vi "MSEncoder Case-22-PhaseScan.vi"(8 "error in (no error)":errorcluster, 9 "ParamValIn":variant, 11 "MSEncoder in":refnum<class "MSEncoder.lvclass">) -> (0 "error out":errorcluster, 3 "MSEncoder out":refnum<class "MSEncoder.lvclass">)   [LabVIEW 2018, in "MSEncoder.lvclass"]
uses:
  MSEncoder.lvclass
  Ctl/MSEditorParam phaseScan.ctl
  PublicSubVI/Ctl/MathieuEqParam.ctl
  MSEncoder.lvclass/MSEncoder.ctl
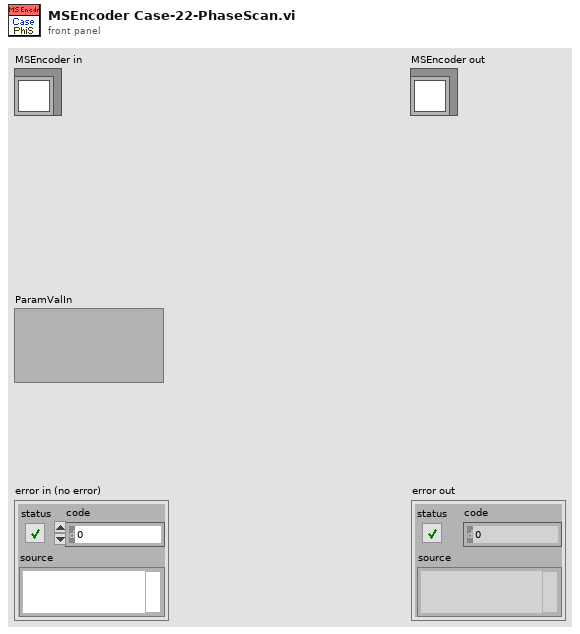
[diagram p1: front panel]
types:
  T1 = typedef "MSEditorParam phaseScan.ctl" = cluster{"auxWfmType":u32, "auxStart":u32, "iauxCyc":ext, "auxCyc":ext, "beta":ext, "betaScale":ext, "auxAmp":ext, "auxPulse1":ext[], "auxPulse2":ext[], "auxPulseAmp":ext[], "time":ext, "freq":ext[], "stepWidth":u32}
  T2 = cluster{"f1":ext, "f2":ext, "Scan Time":ext, "Stepwise":u32}
  T3 = typedef "MathieuEqParam.ctl" = cluster{"mz(Th)":ext, "Amp(V)":ext, "Freq(Hz)":ext, "Beta":ext, "r_0 (mm)":ext, "z_0 (mm)":ext}
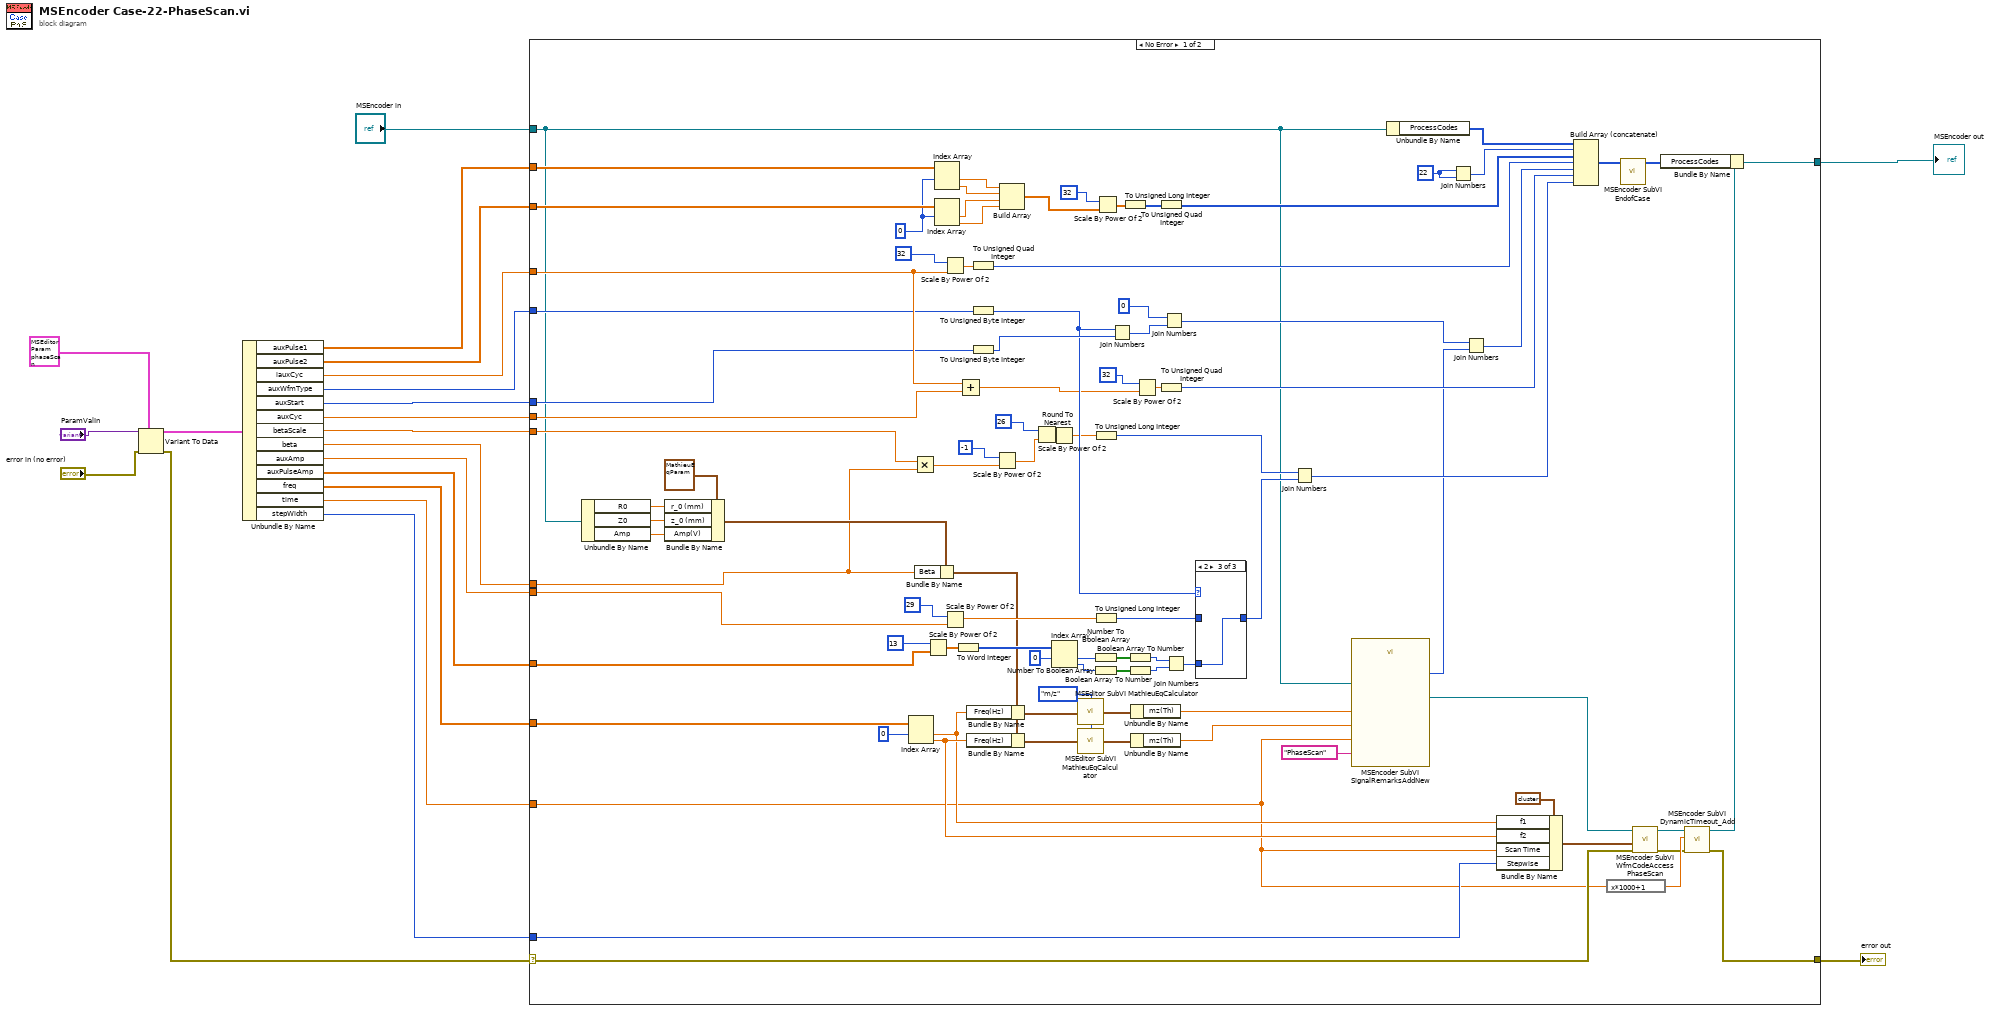
[diagram p0: block diagram]
diagram:
  n1 = Variant To Data(error in="error in (no error)", type=T1 {"auxWfmType"=0, "auxStart"=0, "iauxCyc"=0.0, "auxCyc"=0.0, "beta"=0.5, "betaScale"=1.0, "auxAmp"=1.0, "auxPulse1"=[0.0, 0.5], "auxPulse2"=[0.5, 1.0], "auxPulseAmp"=[1.0, -1.0], "time"=1.0, "freq"=[100000.0, 50000.0], "stepWidth"=1} ("ParamValueType"), Variant="ParamValIn") -> (data=w3:T1, error out=w2:errorcluster)
  n2 = Unbundle By Name(w3) -> ("auxPulse1"=w20:ext[], "auxPulse2"=w19:ext[], "iauxCyc"=w18:ext, "auxWfmType"=w17:u32, "auxStart"=w16:u32, "auxCyc"=w15:ext, "betaScale"=w14:ext, "beta"=w13:ext, "auxAmp"=w12:ext, "auxPulseAmp"=w11:ext[], "freq"=w10:ext[], "time"=w9:ext, "stepWidth"=w8:u32)
  n3 = case shown="No Error" w2 {
    selector: w2 -> [w33 w119]
    tunnel: "MSEncoder in" -> [w36 w118]
    tunnel: [w28 w119] -> w21
    tunnel: [w114 w118] -> w6
    tunnel: w20 -> [w108 _]
    tunnel: w19 -> [w107 _]
    tunnel: w18 -> [w106 _]
    tunnel: w17 -> [w105 _]
    tunnel: w16 -> [w104 _]
    tunnel: w15 -> [w103 _]
    tunnel: w14 -> [w102 _]
    tunnel: w13 -> [w101 _]
    tunnel: w12 -> [w100 _]
    tunnel: w11 -> [w99 _]
    tunnel: w10 -> [w98 _]
    tunnel: w9 -> [w27 _]
    tunnel: w8 -> [w39 _]
    frame No Error {
      w90 = u32 22
      w85 = 0 ("index")
      w93 = enum16{"m/z", "Volt", "Freq", "Beta"}."m/z" ("Target (Freq)")
      n4 = Unbundle By Name(w36) -> ("R0"=w113:ext, "Z0"=w112:ext, "Amp"=w111:ext)
      n5 = Bundle By Name(cluster=T3 {"mz(Th)"=0.0, "Amp(V)"=330.0, "Freq(Hz)"=0.0, "Beta"=1.0, "r_0 (mm)"=10.0, "z_0 (mm)"=7.0710678118654755} ("Parametres in"), "r_0 (mm)"=w113, "z_0 (mm)"=w112, "Amp(V)"=w111) -> (w109:T3)
      n6 = Index Array(array=w98, index #1=0 ("index")) -> (element #1=w37:ext, element #2=w38:ext)  [unwired: 1 in]
      n7 = Multiply(x=w102, y=w101) -> (x*y=w56:ext)
      n8 = Bundle By Name(cluster=w109, "Beta"=w101) -> (w24:T3)
      n9 = Scale By Power Of 2(n=i16 13, x=w99) -> (x*2^n=w54:ext[])
      n10 = Index Array(array=w108, index #1=w85) -> (element #1=w82:ext, element #2=w81:ext)  [unwired: 1 in]
      n11 = Index Array(array=w107, index #1=w85) -> (element #1=w80:ext, element #2=w79:ext)  [unwired: 1 in]
      n12 = Scale By Power Of 2(n=i16 32, x=w106) -> (x*2^n=w87:ext)
      n13 = Scale By Power Of 2(n=i16 29, x=w100) -> (x*2^n=w59:ext)
      n14 = To Word Integer(number=w54) -> (16bit integer=w53:i16[])
      n15 = Add(x=w106, y=w103) -> (x+y=w42:ext)
      n16 = Bundle By Name(cluster=w24, "Freq(Hz)"=w37) -> (w83:T3)
      n17 = Bundle By Name(cluster=w24, "Freq(Hz)"=w38) -> (w97:T3)
      n18 = To Unsigned Quad Integer(1:w87) -> (0:w73:u64)
      n19 = To Unsigned Byte Integer(number=w105) -> (unsigned 8bit integer=w46:u8)
      n20 = To Unsigned Byte Integer(number=w104) -> (unsigned 8bit integer=w72:u8)
      n21 = Scale By Power Of 2(n=i16 -1, x=w56) -> (x*2^n=w62:ext)
      n22 = Build Array(w82, w81, w80, w79) -> (w77:ext[])
      n23 = Scale By Power Of 2(n=i16 26, x=w62) -> (x*2^n=w60:ext)
      n24 = Round To Nearest(number=w60) -> (nearest integer value=w41:ext)
      n25 = Index Array(array=w53, index #1=0 ("index")) -> (element #1=w52:i16, element #2=w51:i16)  [unwired: 1 in]
      n26 = call "MSEditor SubVI MathieuEqCalculator.vi"("Target (Freq)"=w93, "Parametres in"=w83) -> ("Parametres out"=w92:T3)  [unwired: 2 in]
      n27 = call "MSEditor SubVI MathieuEqCalculator.vi"("Target (Freq)"=w93, "Parametres in"=w97) -> ("Parametres out"=w84:T3)  [unwired: 2 in]
      n28 = To Unsigned Long Integer(number=w41) -> (unsigned 32bit integer=w58:u32)
      n29 = To Unsigned Long Integer(number=w59) -> (unsigned 32bit integer=w44:u32)
      n30 = Number To Boolean Array(number=w52) -> (Boolean array=w50:bool[])
      n31 = Number To Boolean Array(number=w51) -> (Boolean array=w49:bool[])
      n32 = Scale By Power Of 2(n=i16 32, x=w77) -> (x*2^n=w76:ext[])
      n33 = Join Numbers(hi=w46, lo=w72) -> ((hi.lo)=w71:u16)
      n34 = To Unsigned Long Integer(number=w76) -> (unsigned 32bit integer=w75:u32[])
      n35 = Boolean Array To Number(Boolean array=w50) -> (number=w47:u16)
      n36 = Boolean Array To Number(Boolean array=w49) -> (number=w48:u16)
      n37 = Unbundle By Name(w92) -> ("mz(Th)"=w23:ext)
      n38 = Unbundle By Name(w84) -> ("mz(Th)"=w22:ext)
      n39 = Scale By Power Of 2(n=i16 32, x=w42) -> (x*2^n=w67:ext)
      n40 = To Unsigned Quad Integer(1:w75) -> (0:w74:u64[])
      n41 = To Unsigned Quad Integer(1:w67) -> (0:w65:u64)
      n42 = Join Numbers(hi=u16 0, lo=w71) -> ((hi.lo)=w69:u32)
      n43 = Join Numbers(hi=w47, lo=w48) -> ((hi.lo)=w45:u32)
      n44 = case shown="2" w46 {
        tunnel: w45 -> [_ _ w117]
        tunnel: w44 -> [w115 w116 _]
        tunnel: [w115 w116 w117] -> w43
        frame 0, Default {
        }
        frame 1 {
        }
        frame 2 {
        }
      }
      n45 = Join Numbers(hi=w58, lo=w43) -> ((hi.lo)=w57:u64)
      n46 = call "MSEncoder SubVI SignalRemarksAddNew.vi"("Label"="PhaseScan", "Scan time"=w27, "mz 1"=w22, "mz 0"=w23, "MSEncoder in"=w36) -> ("Len"=w25:u32, "MSEncoder out"=w34:refnum<class "MSEncoder.lvclass">)  [unwired: 5 in]
      n47 = Unbundle By Name(w36) -> ("ProcessCodes"=w86:u64[])
      n48 = Join Numbers(hi=w90, lo=w90) -> ((hi.lo)=w96:u64)
      n49 = Join Numbers(hi=w69, lo=w25) -> ((hi.lo)=w68:u64)
      n50 = Bundle By Name(cluster=T2 {"f1"=0.0, "f2"=0.0, "Scan Time"=0.0, "Stepwise"=0} ("Phase Data"), "f1"=w37, "f2"=w38, "Scan Time"=w27, "Stepwise"=w39) -> (w35:T2)
      n51 = Build Array (concatenate)(w86, w96, w74, w73, w68, w65, w57) -> (w95:u64[])
      n52 = expression code="x*1000+1"(w27) -> (w30:ext)
      n53 = call "MSEncoder SubVI EndofCase.vi"("Case codes"=w95) -> ("Case codes with end"=w94:u64[])  [unwired: 9 in, 1 out]
      n54 = call "MSEncoder SubVI WfmCodeAccess PhaseScan.vi"("error in"=w33, "Data in"=w35, "MSEncoder in"=w34) -> ("error out"=w29:errorcluster, "MSEncoder out"=w32:refnum<class "MSEncoder.lvclass">)  [unwired: 7 in]
      n55 = call "MSEncoder SubVI DynamicTimeout_Add.vi"("error in (no error)"=w29, "Timeout_ms"=w30, "MSEncoder"=w32) -> ("error out"=w28:errorcluster, "MSEncoder"=w31:refnum<class "MSEncoder.lvclass">)  [unwired: 7 in]
      n56 = Bundle By Name(cluster=w31, "ProcessCodes"=w94) -> (w114:refnum<class "MSEncoder.lvclass">)
    }
    frame Error {
    }
  }
  "error out" <- w21
  "MSEncoder out" <- w6
